vi "ChangeWhileMeasuring.vi"(5 "StopOrRestart":enum16{"StopIfMeasuring", "RestartIfMeasuring"}(ring), 6 "WasMeasuring":bool, 7 "Queue Array In":refnum<queue>[](array[refnum]), 8 "error in (no error)":errorcluster, 11 "ChromaPowerSupplyModel in":refnum<class "ChromaPowerSupplyModel.lvclass">) -> (0 "error out":errorcluster, 3 "ChromaPowerSupplyModel out":refnum<class "ChromaPowerSupplyModel.lvclass">, 4 "WasMeasuring?":bool)   [LabVIEW 2018]
doc: "This VI checks if the instrument is capable of send new instrument setting while the instruments is currently acquiring measurements."
uses:
  AcPwrBaseClass/AcPwrBase.lvclass
  Common/clMessage.ctl
  AcPwrPlugins.lvlib
  ChromaPowerSupplyModel.lvclass
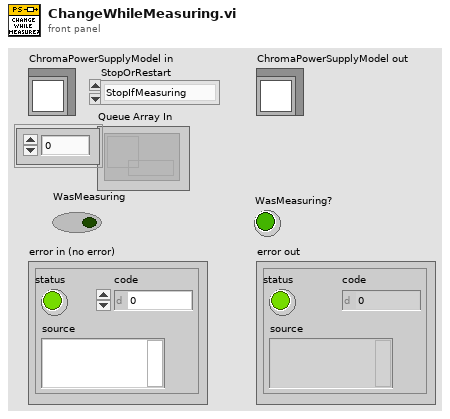
[diagram p1: front panel]
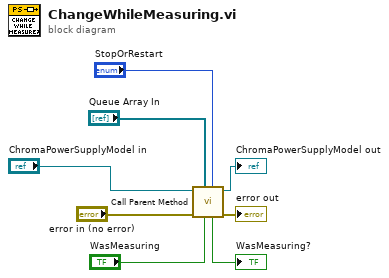
[diagram p0: block diagram]
diagram:
  n1 = call-parent "Call Parent Method"("StopOrRestart"="StopOrRestart", "WasMeasuring"="WasMeasuring", "Queue Array In"="Queue Array In", "error in (no error)"="error in (no error)", "AcPwrBase in"="ChromaPowerSupplyModel in") -> ("error out"=→"error out":errorcluster, "AcPwrBase out"=→"ChromaPowerSupplyModel out":refnum<class "ChromaPowerSupplyModel.lvclass">, "WasMeasuring?"=→"WasMeasuring?":bool)  [unwired: 4 in]
